vi "EventLog.File.ReadWrite.vi"(6 "read count (ALL)":i32=-1, 7 "action (read)":enum16{"read", "write"}(ring), 8 "error in":errorcluster, 9 "read offset (in bytes)":i64, 10 "Events in":T1[](array[typedef]) {"ts" format="%<%X\n%x>T"}, 11 "file":path) -> (0 "error out":errorcluster, 1 "offset (in bytes)":i64, 2 "Events out":T1[](array[typedef]) {"ts" format="%<%X\n%x>T"}, 3 "size (in bytes)":i64, 4 "End of File?":bool)   [LabVIEW 2016]
uses:
  EventLog.Event.ctl
  EventLog.EventLevel.ctl
  EventLog.EventSource.ctl
  Translator/Translator.Message.ctl
  Global/ApplicationGlobal.vi
panel:
  out "size(s)":i32
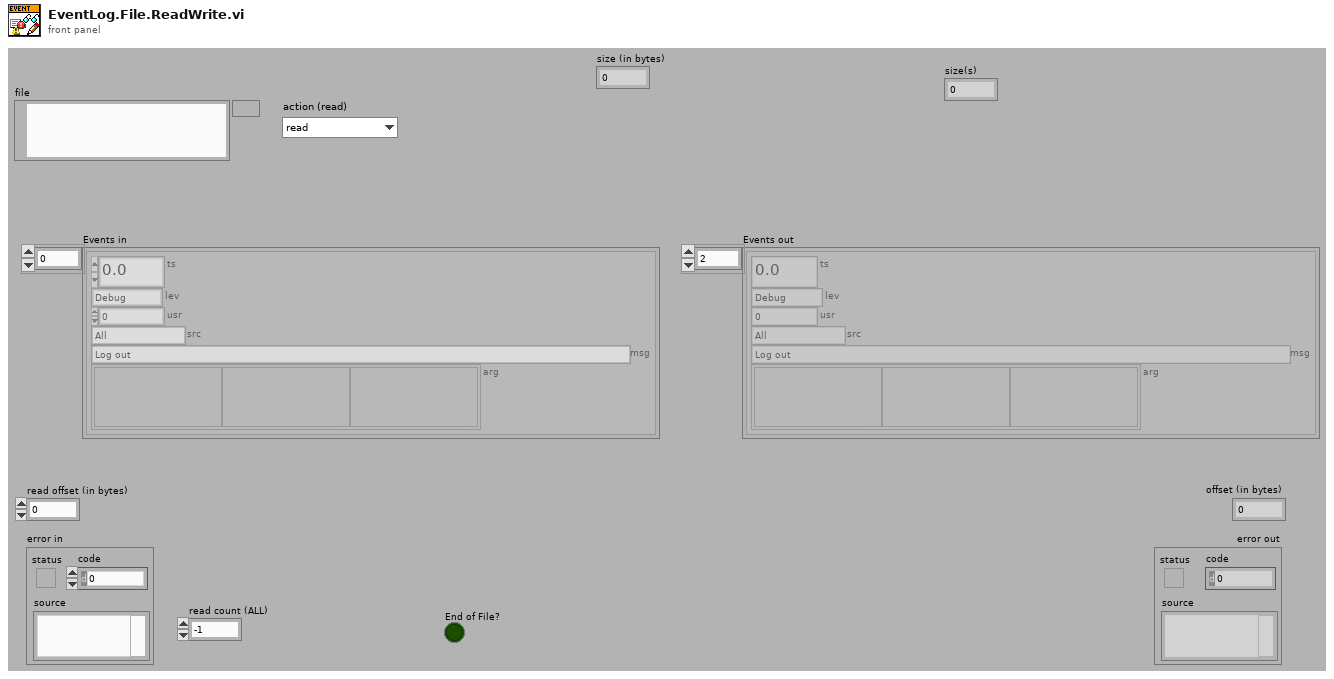
[diagram p1: front panel]
types:
  T1 = typedef "EventLog.Event.ctl" = cluster{"ts":dbl, "lev":T2, "usr":i32, "src":T3, "msg":T4, "arg":variant[]}
  T2 = typedef "EventLog.EventLevel.ctl" = enum8{"Debug", "Info", "Warning", "Error"}
  T3 = typedef "EventLog.EventSource.ctl" = enum16{"All", "Gui", "Ref", "File", "Arch", "Seq", "CPX", "DB", "Laser", "Scan.P", "Scan.O"}
  T4 = typedef "Translator.Message.ctl" = enum16{"-", "Event confirmed", "Log out", "Log in", "Shutdown", "Cancel", "Start", "Begin time", "End time", "Duration", "Service Mode", "Ignore Results", "Serial Format", "On", "Off", "OK", "NOK", "NOK %s", "Home", "Work", "Close", "Open", "In progress...", "Missing", "Empty", "Hardware failure", "Initial", "Default", "Total", "Out of range", "Free disk space is below 1GB - contact technician", "Error %d >> %s", "Error %d >> %s >> %s", "Msg %d >> %s", "Laser msg %d %s", "Laser cmd error %s %d", "Laser cmd failed %s", "Laser cmd warning %s", "Laser disconnected", "Laser status %s", "Laser already started", "Laser job unkonwn %s", "Laser job missing %s", "Laser job select failure %s", "Unable to start laser printing (%s)", "Unable to stop laser printing (%s)", "Laser marking aborted", "Laser marking timeout", "Unable to reset Laser Interlock (%s)", "Unable to trigger Laser. Laser not ready (%s)", "Laser job '%s' coordinates not configured", "Starting %s", "Quitting %s", "Configured", "Initializing", "Quitting", "Loading", "Loaded %d results", "Loaded %d events", "Running", "Stopped", "Summary", "Laser", "Do you want to continue?", "Do you want to delete the configuration?", "The configuration is being used by an order. Unable to delete!", "Press confirm button", "Station is not based. Do you want to exit?", "Station requires changeover. Do you want to run the test?", "Test options are not set as default. Do you want to continue?", "Formatting of WabcoNo is disabled. Do you want to continue?", "Product not detected. Do you want to continue?", "Product scan failed. Do you want to continue?", "Calibration", "Log out?", "System", "All", "IDLE", "Translating...%s", "Not found", "Alarm %s", "Run", "Skip", "Abort", "Repeat", "Please wait...", "Database disconnected", "Database disconnected - changeover disabled!", "Login to database successful", "Login to database failed: %d; %s", "Unable to check the product status of reference %d - database disconnected", "Unable to set the product status of reference %d - database disconnected", "Variant file backup %s", "Read variant (%s)", "Result", "Station armed!", "Station requires changeover!", "Select reference number...", "EMERGENCY BUTTON - press Control button", "EMERGENCY DOOR - press Control button", "Resetting Emergency...", "Unable to reset safety circuit - Emergency Button pressed", "Unable to reset safety circuit - Emergency Side Door open", "Station not based", "Station based", "Station not empty", "Station basing...", "No order", "Press Start to begin new order", "Scanning new order", "Order NOK. Correct or scan again", "Order OK. Press Accept", "Order ready", "Revolver incorrect", "Fork incorrect", "Revolver missing", "Revolver empty", "Container missing", "Offline results", "Offline statistics", "Updating statistics %.1f %%", "DMC Configurator", "Door open", "Close the front door", "Press start button", "Done. Open the front door", "Running...", "Running...%.1f %%", "Pause %s", "Pause %s. NOK container missing", "Pause %s. OK container missing", "Pause %s. Revolver empty", "Pause %s. Revolver missing", "Pause %s. Revolver incorrect", "Pause %s. Fork missing", "Pause %s. Fork incorrect", "Pause %s. Too many failures", "Pause %s. Unloading failure", "Pause %s. One slot is not working", "Pause %s. Part order is done. Empty OK container", "Pause %s. Unable to move product to slot", "Pause %s. Unable to move back product pusher", "Pause %s. Unable to lift product", "Pause %s. Unable to move back product lifter", "Pause %s. Unable to move product arm to Work", "Pause %s. Unable to move product arm to NOK", "Pause %s. Unable to move product arm to OK", "Pause %s. Unable to unsuck the NOK product", "Pause %s. Unable to drop the NOK product", "Pause %s. Product OK missing", "Pause %s. Unable to unsuck the OK product", "Pause %s. Unable to drop the OK product", "Stopping...", "File '%s' is missing", "File '%s' is broken", "File '%s' is running", "Log file started (%s)", "Log file ended (%s)", "Log file stopped (%s)", "Log file ignored (%s)", "Log file exported (%s)", "Log file export failed (%s)", "Wrong serial number in log file", "Wrong reference number in log file", "Test steps are missing", "%s = %.3f", "Process param '%s' not found in DB", "Process param '%s' wrong order", "Process param '%s' value %.3f out of limits (%.3f; %.3f)", "Step%d param '%s' not found in DB", "Step%d param '%s' wrong order", "Step%d param '%s' value %.3f out of limits (%.3f; %.3f)", "Step%d EV '%s' not found in DB", "Step%d EV '%s' wrong order", "\"%s\" not found in DB", "\"%s\" wrong order", "\"%s\" value %.3f out of limits (%.3f; %.3f)", "\"%s\" not found in software", "Process init (%s)", "Process started", "Process restarted", "Process run", "Process done", "Process done - remove OK container", "Process aborted", "Process aborted at work", "Process aborted at home", "Process error", "Process error at home", "Process error at work", "Process close", "Process pause", "Process continue", "Process door open", "Process door close", "Process pause at slot %s due to %s", "Select plate from the order to process", "Do you want to start the process?", "Do you want to continue the process?", "There is unfinished order. Do you want to put the new order?", "Product %s %d OK", "Product %s %d NOK", "Unable to unload the slot %s. Product missing in the slot", "Unable to unload the slot %s. Product already in the arm", "Unable to accept the product as OK. Product missing in slot %s", "Unable to accept the product as OK. Product could not drop into the container at slot %s", "Unable to accept the product as NOK. Product could not drop into the container at slot %s", "Scan failed. Error %s", "Scan failed. Scanner disconnected", "Scan failed. Wrong Wabco number %d, limit (%d,%d)", "Scan failed. Wrong serial number %d, limit (%d,%d)", "Scan failed. Wrong date %d, limit (%d,%d)", "Scan failed. Wrong product wabco number %d (expected %d)", "Scan failed. Wrong product serial number %d (expected > 0)", "Scan OK %s", "Scan failed. Unable to determine table position (%s)", "Scan failed. Timeout", "Tune failed. Scanner disconnected", "Tune failed. Timeout", "%s = %d", "%s = %d->%d", "Unable to set %s = %.2f - Air Pressure Inside off", "Unable to set digital output '%s' = %d", "Unable to activate air pressure inside - timeout", "Unable to activate air pressure inside - aborted", "Unable to switch on Air Main Valve - Air Pressure Inlet off", "Unable to switch on Air Main Valve - Door open", "Unable to switch off Air Main Valve - timeout", "Unable to switch off Air Main Valve - aborted", "Unable to rotate Table - timeout", "Unable to rotate Table - aborted", "Unable to rotate Table - Product Move not in Home position", "Unable to rotate Table - Air Pressure Inside off", "Unable to rotate Table - Product Lift A not in Home position", "Unable to rotate Table - Product Lift B not in Home position", "Unable to rotate Table - unlock before movement timeout", "Unable to rotate Table - lock after movement timeout", "Unable to move Table Lock to %s position - timeout", "Unable to move Table Lock to %s position - aborted", "Unable to move Table Lock to %s position - Air Pressure Inside off", "Unable to move Table Lock to %s position - Table not in position", "Unable to move Product Lift A to %s position - timeout", "Unable to move Product Lift B to %s position - timeout", "Unable to move Product Lift A to %s position - aborted", "Unable to move Product Lift B to %s position - aborted", "Unable to move Product Lift A to %s position - Air Pressure Inside off", "Unable to move Product Lift B to %s position - Air Pressure Inside off", "Unable to move Product Lift A to %s position - Table not locked", "Unable to move Product Lift B to %s position - Table not locked", "Unable to move Product Lift A to %s position - Product Arm not in Work position", "Unable to move Product Lift B to %s position - Product Arm not in Work position", "Unable to set Product Suction Gripper %s to %s - timeout", "Unable to set Product Suction Gripper %s to %s - aborted", "Unable to set Product Suction Gripper %s to %s - Air Pressure Inside off", "Unable to set Product Suction Gripper %s to %s - Table slot unkown", "Unable to move Product Arm to %s position - timeout", "Unable to move Product Arm to %s position - aborted", "Unable to move Product Arm to %s position - Air Pressure Inside off", "Unable to move Product Arm to %s position - Product Lift A not in Home position", "Unable to move Product Arm to %s position - Product Lift B not in Home position", "Unable to move Product to %s position - timeout", "Unable to move Product to %s position - aborted", "Unable to move Product to %s position - Air Pressure Inside off", "Unable to move Product to %s position - Table not in position"}
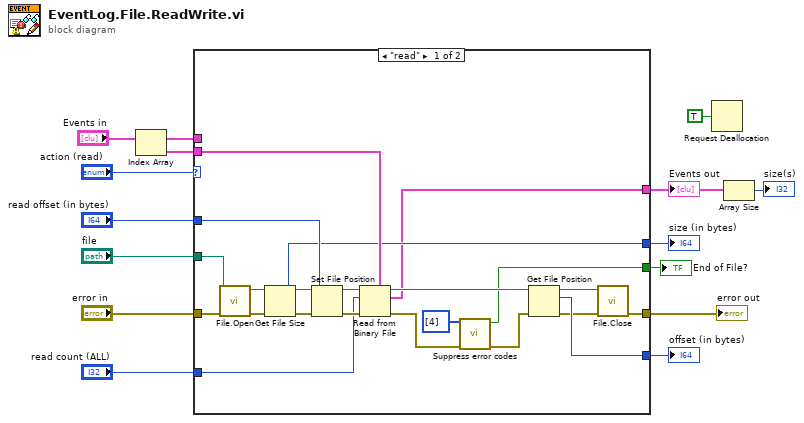
[diagram p0: block diagram]
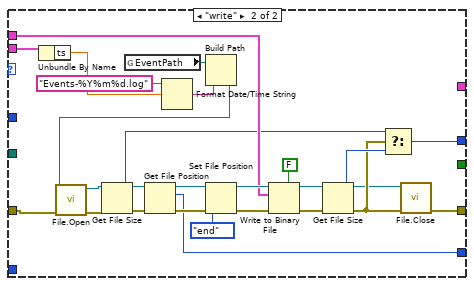
[diagram p2: hidden frame]
diagram:
  n1 = Index Array(array="Events in") -> (element=w4:T1)  [unwired: 1 in]
  n2 = case shown="\"read\"" "action (read)" {
    tunnel: [w24 w49] -> w7
    tunnel: "error in" -> [w18 w43]
    tunnel: "Events in" -> [_ w53]
    tunnel: "read offset (in bytes)" -> [w23 _]
    tunnel: [w15 _] -> w10
    tunnel: "read count (ALL)" -> [w30 _]
    tunnel: [w27 w58] -> w11
    tunnel: [w20 w56] -> w8
    tunnel: [w31 _] -> w6
    tunnel: w4 -> [w28 w39]
    tunnel: "file" -> [w16 _]
    frame "read" {
      n3 = call "File.Open.vi"("error in"=w18, "file"=w16) -> ("error out"=w19:errorcluster, "File ref out"=w17:refnum<file>)  [unwired: 8 in]
      n4 = Get File Size(file=w17, error in=w19) -> (refnum out=w22:refnum<file>, size (in bytes)=w20:i64, 0:w21:errorcluster)
      n5 = Set File Position(offset (in bytes) (0)=w23, refnum=w22, error in=w21) -> (refnum out=w35:refnum<file>, error out=w36:errorcluster)  [unwired: 1 in]
      n6 = Read from Binary File(5:w28, 8:w36, 10:w30, 11:w35) -> (0:w29:errorcluster, 2:w15:T1[], 3:w34:refnum<file>)  [unwired: 2 in, 1 out]
      n7 = call "Suppress error codes.vi"("error in (no error)"=w29, "suppress codes([43])"=i32[] [4]) -> ("error out"=w32:errorcluster, "suppressed"=w31:bool)  [unwired: 8 in]
      n8 = Get File Position(4:w32, 7:w34) -> (0:w25:errorcluster, 2:w27:i64, 3:w26:refnum<file>)
      n9 = call "File.Close.vi"("error in"=w25, "File ref in"=w26) -> ("error out"=w24:errorcluster)  [unwired: 9 in]
    }
    frame "write" {
      n10 = Unbundle By Name(w39) -> ("ts"=w38:dbl)
      n11 = global read "ApplicationGlobal.vi" "EventPath"() -> (w41:path)
      n12 = Format Date/Time String(time format string (%c)="Events-%Y%m%d.log", seconds (now)=w38) -> (date/time string=w40:string)  [unwired: 1 in]
      n13 = Build Path(base path=w41, name or relative path=w40) -> (appended path=w37:path)
      n14 = call "File.Open.vi"("error in"=w43, "file"=w37) -> ("error out"=w45:errorcluster, "File ref out"=w44:refnum<file>)  [unwired: 8 in]
      n15 = Get File Size(file=w44, error in=w45) -> (refnum out=w48:refnum<file>, size (in bytes)=w46:i64, 0:w47:errorcluster)
      n16 = Get File Position(4:w47, 7:w48) -> (0:w60:errorcluster, 2:w58:i64, 3:w59:refnum<file>)
      n17 = Set File Position(refnum=w59, from (0:start)=enum16{"start", "end", "current"}."end", error in=w60) -> (refnum out=w63:refnum<file>, error out=w62:errorcluster)  [unwired: 1 out]
      n18 = Write to Binary File(file (use dialog)=w63, data=w53, error in=w62, 5:FALSE ("prepend array or string size? (T)")) -> (refnum out=w55:refnum<file>, error out=w54:errorcluster)  [unwired: 2 in, 1 out]
      n19 = Get File Size(file=w55, error in=w54) -> (refnum out=w50:refnum<file>, size (in bytes)=w57:i64, 0:w51:errorcluster)
      n20 = Select(t=w46, s=w51, f=w57) -> (s? t:f=w56:i64)
      n21 = call "File.Close.vi"("error in"=w51, "File ref in"=w50) -> ("error out"=w49:errorcluster)  [unwired: 9 in]
    }
  }
  "error out" <- w7
  "Events out" <- w10
  "offset (in bytes)" <- w11
  "size (in bytes)" <- w8
  "End of File?" <- w6
  n22 = Request Deallocation(TRUE ("flag")) -> ()
  n23 = Array Size(array=w10) -> (size(s)=→"size(s)":i32)
